vi "报警信息.vi"(8 "error in (no error)":errorcluster, 11 "报警信息":string) -> (0 "error out":errorcluster)   [LabVIEW 2016, in "斯坦道多参数.lvlib"]
uses:
  <vilib>/Utility/sysdir.llb/System Directory Type.ctl
  <vilib>/addons/database/Connection.llb/DB Tools Open Connec (String).vi
  <vilib>/addons/database/NI_Database_API.lvlib
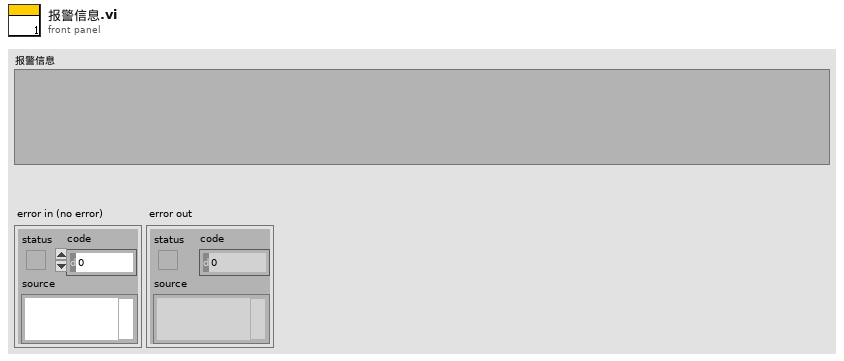
[diagram p1: front panel]
types:
  T1 = cluster{"时间标识":timestamp, "设备":string, "报警信息":string}
  T2 = typedef "System Directory Type.ctl" = i32
  T3 = typedef "NI_Database_API.lvlib/Conn ObjectReference.ctl" = refnum<k1>
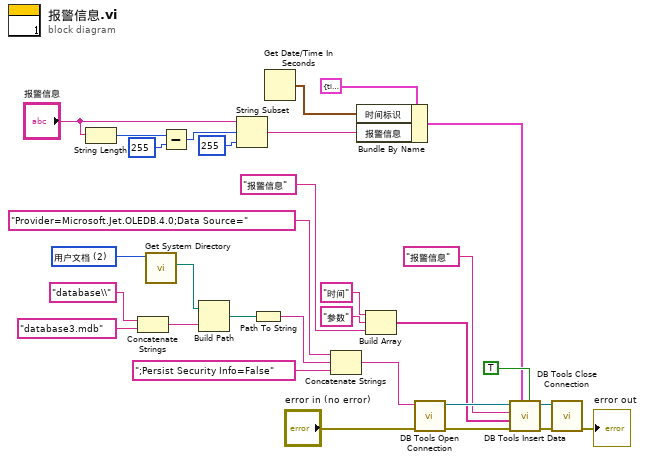
[diagram p0: block diagram]
diagram:
  w25 = T2 2 items=["用户目录"=0, "用户桌面"=1, "用户文档"=2, "用户应用程序数据"=3, "用户设置"=4, "用户临时目录"=5, "公共文档"=6, "公共应用程序数据"=7, "公共设置"=8, "公共缓存"=13, "系统核心库"=9, "系统安装库"=10, "应用程序文件"=11, "启动盘根目录"=12] ("system directory type")
  n1 = String Length(string="报警信息") -> (length=w4:i32)
  n2 = Concatenate Strings("database\\" ("condition"), "database3.mdb" ("database")) -> (w17:string)
  n3 = call <vilib>:"Get System Directory.vi"("system directory type"=w25) -> ("system directory"=w23:path)  [unwired: 10 in]
  n4 = Subtract(x=w4, y=255 ("长度（剩余）")) -> (x-y=w2:i32)
  n5 = Build Path(base path=w23, name or relative path=w17) -> (appended path=w22:path)
  n6 = String Subset(string="报警信息", offset (0)=w2, length (rest)=255 ("长度（剩余）")) -> (substring=w1:string)
  n7 = Path To String(path=w22) -> (string=w21:string)
  n8 = Get Date/Time In Seconds() -> (seconds since 1Jan1904=w10:timestamp)
  n9 = Concatenate Strings("Provider=Microsoft.Jet.OLEDB.4.0;Data Source=" ("condition"), w21, ";Persist Security Info=False" ("condition")) -> (w19:string)
  n10 = Bundle By Name(cluster=T1 {"时间标识"=timestamp(0 s since 1904-01-01), "设备"="多参数", "报警信息"=""} ("data in"), "时间标识"=w10, "报警信息"=w1) -> (w9:T1)
  n11 = Build Array("时间", "参数" ("元素"), "报警信息") -> (w13:string[])
  n12 = call-poly <vilib>:"DB Tools Open Connection.vi"("error in (no error)"="error in (no error)", "connection information"=w19) -> ("error out"=w15:errorcluster, "connection reference"=w16:T3)  [unwired: 6 in]
  n13 = call <vilib>:"DB Tools Insert Data.vi"("create table? (F)"=TRUE, "data"=w9, "error in (no error)"=w15, "columns"=w13, "table"="报警信息", "connection reference"=w16) -> ("error out"=w27:errorcluster, "connection reference out"=w28:T3)  [unwired: 4 in]
  n14 = call <vilib>:"DB Tools Close Connection.vi"("error in (no error)"=w27, "connection reference"=w28) -> ("error out"=→"error out":errorcluster)  [unwired: 5 in]
